vi "DAQmx Create Channel (AI-Voltage-RMS).vi"(0 "task in":refnum<k21>, 1 "maximum value":dbl=5.0 format="%0.2f", 2 "minimum value":dbl=-5.0 format="%0.2f", 3 "input terminal configuration":i32(ring)=-1 items=["default"=-1, "RSE"=10083, "NRSE"=10078, "Differential"=10106, "Pseudodifferential"=12529], 5 "physical channels":tag, 7 "name to assign":string, 9 "units":i32(ring)=10348 items=["Volts"=10348, "From Custom Scale"=10065], 11 "error in":errorcluster, 12 "custom scale name":tag) -> (4 "task out":refnum<k21>, 15 "error out":errorcluster)   [LabVIEW 2011]
doc: "Creates channel(s) to measure voltage RMS, the average (mean) power of the acquired voltage."
uses:
  C:/Program Files/National Instruments/LabVIEW 2011/resource/objmgr/daqmx.rc
panel:
  # "input limits"
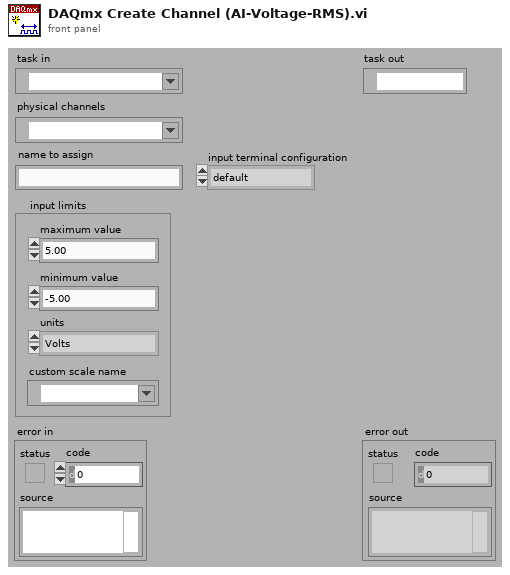
[diagram p1: front panel]
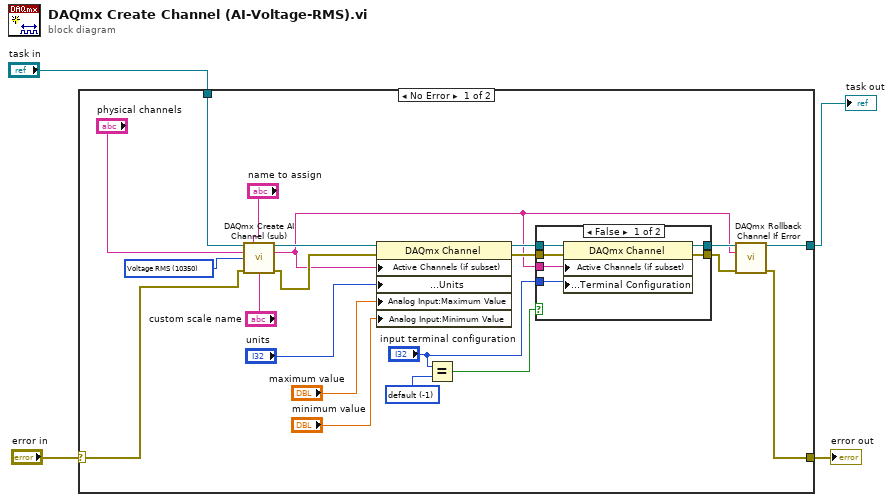
[diagram p0: block diagram]
diagram:
  n1 = case shown="No Error" "error in" {
    selector: "error in" -> [w24 w35]
    tunnel: [w7 w35] -> w2
    tunnel: "task in" -> [w25 w34]
    tunnel: [w8 w34] -> w1
    frame No Error {
      w5 = 10350 items=["Voltage"=10322, "Voltage RMS"=10350, "Current"=10134, "Current RMS"=10351, "More:Voltage:Custom with Excitation"=10323, "Frequency"=10181, "Resistance"=10278, "Temperature:Thermocouple"=10303, "Temperature:Thermistor"=10302, "Temperature:RTD"=10301, "Temperature:Built-in Sensor"=10311, "Strain Gage"=10300, "Position:LVDT"=10352, "Position:RVDT"=10353, "Accelerometer"=10356, "Sound Pressure:Microphone"=10354, "TEDS Sensor"=12531] ("AI.MeasType")
      w14 = -1 items=["default"=-1, "differential"=10106, "RSE"=10083, "NRSE"=10078] ("input terminal configuration")
      n2 = call "DAQmx Create AI Channel (sub).vi"("task in"=w25, "virtual channel name"="name to assign", "physical channel name"="physical channels", "measurement type"=w5, "error in"=w24, "custom scale"="custom scale name") -> ("task out"=w11:refnum<k21>, "channel names"=w6:string, "error out"=w21:errorcluster)  [unwired: 1 in, 6 out]
      n3 = property class="DAQmx Channel"(reference=w11, error in=w21, "Active Channels (if subset)"=w6, "Analog Input:Voltage:AC RMS Voltage:Units"="units", "Analog Input:Maximum Value"="maximum value", "Analog Input:Minimum Value"="minimum value") -> (reference out=w12:refnum<k21>, error out=w17:errorcluster)
      n4 = Equal?(x="input terminal configuration", y=w14) -> (x = y?=w18:bool)
      n5 = case shown="False" w18 {
        tunnel: w17 -> [w31 w33]
        tunnel: [w30 w32] -> w10
        tunnel: [w29 w33] -> w9
        tunnel: "input terminal configuration" -> [w28 _]
        tunnel: w6 -> [w27 _]
        tunnel: w12 -> [w26 w32]
        frame False {
          n6 = property class="DAQmx Channel"(reference=w26, error in=w31, "Active Channels (if subset)"=w27, "Analog Input:General Properties:Input Configuration:Terminal Configuration"=w28) -> (reference out=w30:refnum<k21>, error out=w29:errorcluster)
        }
        frame True {
        }
      }
      n7 = call "DAQmx Rollback Channel If Error.vi"("task in"=w10, "channel names"=w6, "error in"=w9) -> ("task out"=w8:refnum<k21>, "error out"=w7:errorcluster)  [unwired: 11 out]
    }
    frame Error {
    }
  }
  "error out" <- w2
  "task out" <- w1
